vi "dinkdonk.vi"() -> ()   [LabVIEW 2020]
uses:
  <vilib>/MakerHub/LINX/Private/Device/Type Defs/Stimulus Pulse.ctl
  <vilib>/MakerHub/LINX/Public/Peripherals/Analog/Analog Read 1 Chan.vi
  <vilib>/MakerHub/LINX/Public/Peripherals/Digital/Digital Write 1 Chan.vi
  <vilib>/MakerHub/LINX/Public/Peripherals/PWM/PWM Set Duty Cycle 1 Chan.vi
  <vilib>/MakerHub/LINX/Public/Peripherals/Analog/Analog Read N Chans.vi
  <vilib>/MakerHub/LINX/Public/Peripherals/Digital/Digital Write N Chans.vi
  <vilib>/MakerHub/LINX/Private/Local IO/LinxAnalogRead.vi
  <vilib>/MakerHub/LINX/Public/Utilities/Check Channel.vi
  <vilib>/MakerHub/LINX/Private/Local IO/LinxDigitalWrite.vi
  <vilib>/MakerHub/LINX/Public/Utilities/Open Serial.vi
  <vilib>/MakerHub/LINX/Private/Utilties/Generate Error.vi
  <vilib>/MakerHub/LINX/Public/Peripherals/PWM/PWM Set Duty Cycle N Chans.vi
  <vilib>/MakerHub/LINX/LMH-LINX.lvlib
  <vilib>/MakerHub/LINX/Private/Device/Device.lvlib
panel:
  in  "Knob 2":dbl(knob) scale=0.0..1.0
  in  "Echo":u8
  in  "Trigger":u8
  out "Waveform Chart":dbl(graph)
  out "Distance(cm)":u32
  out "Pulse Width (uS)":u32
  in  "stop":bool
  out "x*y":dbl
  out "voltage across ldr":dbl
  in  "Knob":dbl(knob) scale=0.0..1.0
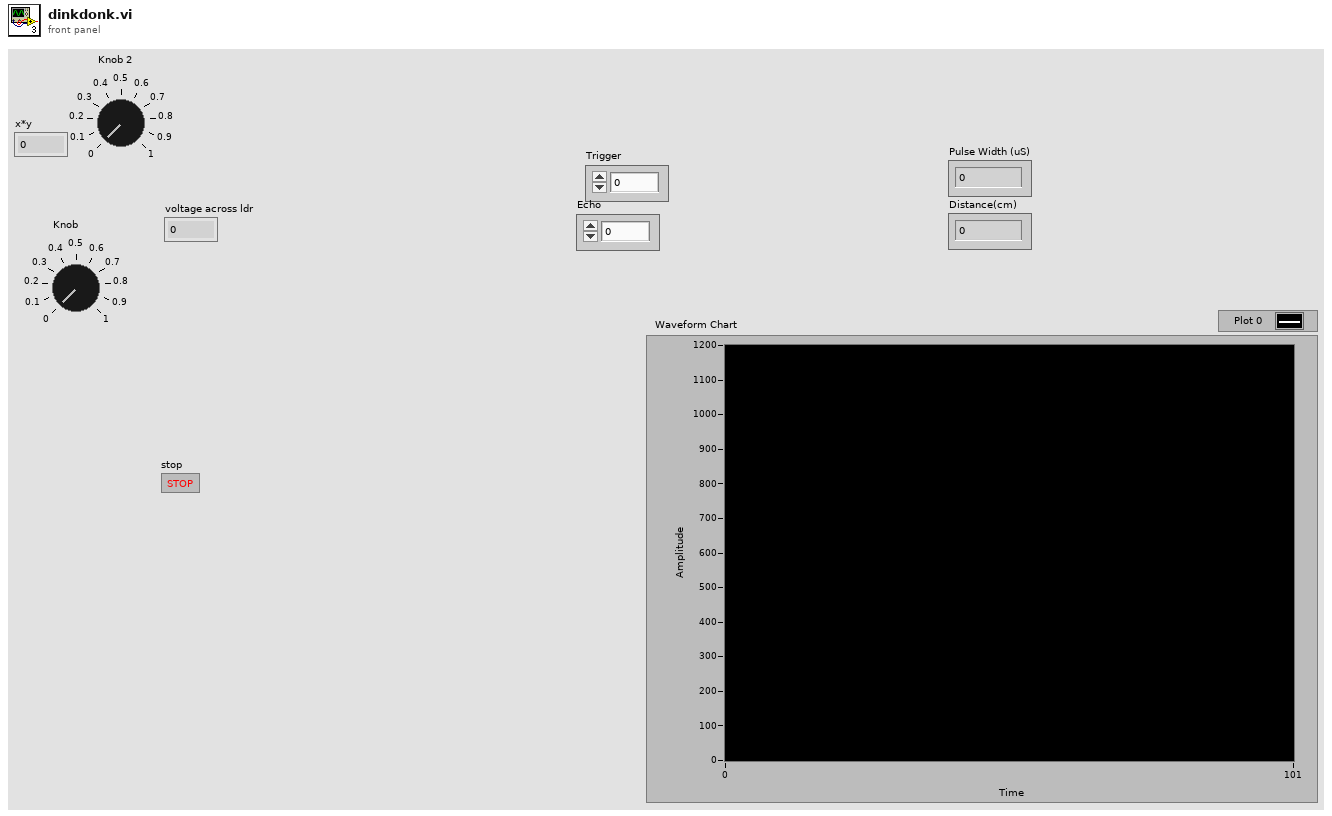
[diagram p1: front panel]
types:
  T1 = typedef "LMH-LINX.lvlib/LINX Ref.ctl" = cluster{"IO":T2, "Interface":T3, "LINX Device Config":T4}
  T2 = typedef "LMH-LINX.lvlib/Platform.ctl" = enum16{"Remote", "Local"}
  T3 = typedef "LMH-LINX.lvlib/Interface.ctl" = enum16{"Serial", "TCP"}
  T4 = typedef "LMH-LINX.lvlib/Device.lvlib/LINX Device Config.ctl" = cluster{"Interface":T3, "COM Port":refnum<visa-resource-name>, "TCP Configuration":T5, "Device Family":u8, "Device ID":u8, "Device Name":string, "TCP Ref":refnum<k5>, "Channels":T6}
  T5 = typedef "LMH-LINX.lvlib/Device.lvlib/TCP Config.ctl" = cluster{"IP Address":string, "Port":u16}
  T6 = typedef "LMH-LINX.lvlib/Channels.ctl" = cluster{"DI":u8[], "DO":u8[], "AI":u8[], "AO":u8[], "PWM":u8[], "QE":u8[], "UART":u8[], "I2C 2":u8[], "SPI":u8[], "CAN":u8[], "Servo":u8[], "AI Ref (V)":dbl, "AI Resolution (Bits)":u8, "AO Ref (V)":dbl, "AO Resolution (Bits)":u8}
  T7 = typedef "LMH-LINX.lvlib/Device.lvlib/Stimulus Pulse.ctl" = enum16{"None", "Active Low", "Active High"}
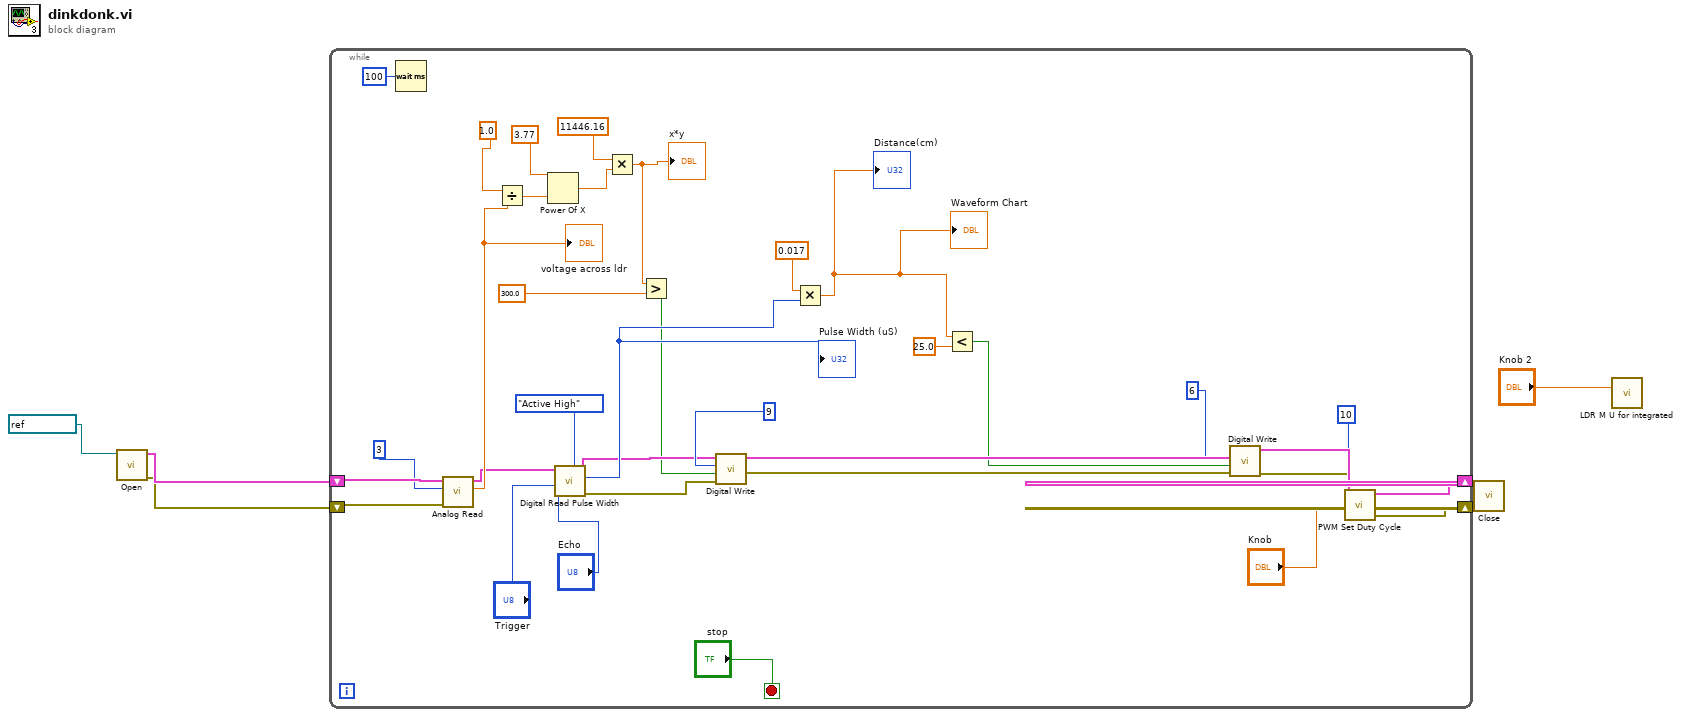
[diagram p0: block diagram]
diagram:
  n1 = call-poly <vilib>:"Open.vi"("Serial Port"=refnum<visa-resource-name> "COM15") -> ("Error Out"=w5:errorcluster, "LINX Resource"=w6:T1)  [unwired: 8 in, 1 out]
  n2 = while {
    shift-right: [w15] -> w4
    shift-left: w6 -> [w41]
    shift-right: [w14] -> w3
    shift-left: w5 -> [w40]
    stop <- "stop" stop-if-true
    n3 = Wait (ms)(milliseconds to wait=u32 100) -> ()  [unwired: 1 out]
    n4 = call-poly <vilib>:"Analog Read.vi"("Error In"=w40, "Analog Channel"=u8 3, "LINX Resource"=w41) -> ("Voltage"=w31:dbl, "LINX Resource"=w13:T1)  [unwired: 5 in, 2 out]
    "voltage across ldr" <- w31
    n5 = Divide(x=1.0, y=w31) -> (x/y=w35:dbl)
    n6 = Power Of X(1:w35, 2:3.77 ("y")) -> (0:w33:dbl)
    n7 = call <vilib>:"Digital Read Pulse Width.vi"("Stimulus Pulse (Active High)"=Stimulus_Pulse."Active High", "DO Channel"="Trigger", "DI Channel"="Echo", "LINX Resource"=w13) -> ("Error Out"=w11:errorcluster, "Pulse Width (uS)"=w20:u32, "LINX Resource"=w12:T1)  [unwired: 5 in]
    "Pulse Width (uS)" <- w20
    n8 = Multiply(x=11446.16, y=w33) -> (x*y=w8:dbl)
    "x*y" <- w8
    n9 = Greater?(x=w8, y=300.0) -> (0:w9:bool)
    n10 = call-poly <vilib>:"Digital Write.vi"("Error In"=w11, "Output Value"=w9, "DO Channel"=u8 9, "LINX Resource"=w12) -> ("Error Out"=w23:errorcluster, "LINX Resource"=w29:T1)  [unwired: 6 in]
    n11 = Multiply(x=0.017, y=w20) -> (x*y=w19:dbl)
    "Distance(cm)" <- w19
    "Waveform Chart" <- w19
    n12 = Less?(x=w19, y=25.0) -> (x < y?=w10:bool)
    n13 = call-poly <vilib>:"Digital Write.vi"("Error In"=w23, "Output Value"=w10, "DO Channel"=u8 6, "LINX Resource"=w29) -> ("Error Out"=w26:errorcluster, "LINX Resource"=w27:T1)  [unwired: 6 in]
    n14 = call-poly <vilib>:"PWM Set Duty Cycle.vi"("Error In"=w26, "Duty Cycle (0-1)"="Knob", "PWM Channel"=u8 10, "LINX Resource"=w27) -> ("Error Out"=w14:errorcluster, "LINX Resource"=w15:T1)  [unwired: 6 in]
  }
  n15 = call <vilib>:"Close.vi"("Error In"=w3, "LINX Resource"=w4) -> ()  [unwired: 9 in, 1 out]
  n16 = call "LDR M U for integrated.vi"("Knob"="Knob 2") -> ()  [unwired: 21 in, 6 out]
